vi "IO Name to Enable Line.vi"(8 "error in (no error)":errorcluster, 10 "IO Name":string, 11 "RIO Target in":refnum<class "RIO Target.lvclass">) -> (0 "error out":errorcluster, 2 "Enable Line":string, 3 "RIO Target out":refnum<class "RIO Target.lvclass">)   [LabVIEW 2014, in "RIO Target.lvclass"]
uses:
  RIO Target.lvclass
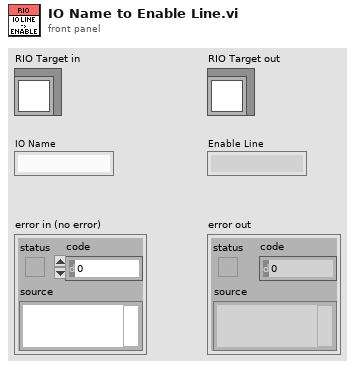
[diagram p1: front panel]
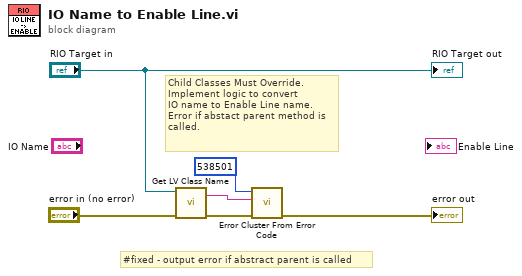
[diagram p0: block diagram]
diagram:
  # "#fixed - output error if abstract parent is called"
  # "Child Classes Must Override.\nImplement logic to convert \nIO name to Enable Line name.\nError if abstact parent method is\ncalled."
  n1 = call <vilib>:"Get LV Class Name.vi"("error in (no error)"="error in (no error)", "object"="RIO Target in") -> ("error out"=w4:errorcluster, "class name"=w3:string)  [unwired: 8 in]
  n2 = call <vilib>:"Error Cluster From Error Code.vi"("error in (no error)"=w4, "error message (\"\")"=w3, "error code (0)"=538501) -> ("error out"=→"error out":errorcluster)  [unwired: 6 in]
  "RIO Target out" <- "RIO Target in"
